vi "add.vi"() -> ()   [LabVIEW 2017]
panel:
  out "error out":errorcluster
  out "Result":string="Popsicle"
  out "x+y":i32
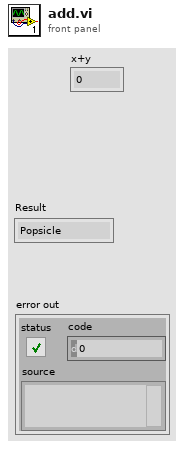
[diagram p1: front panel]
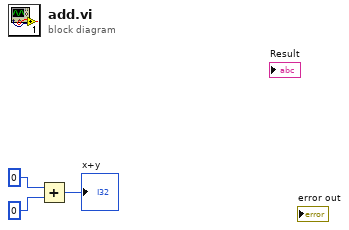
[diagram p0: block diagram]
diagram:
  n1 = Add(x=0, y=0) -> (x+y=→"x+y":i32)
